vi "Read Counter Input PWM Module.vi"   [LabVIEW 2017, in "Scan Engine Scripting.lvlib"]
uses:
  Scan Engine Scripting.lvlib
  NI 9423/NI 9423.lvclass
  NI 9437/NI 9437.lvclass
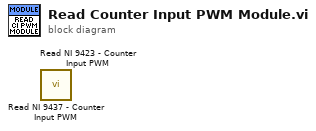
[diagram p0: block diagram]
diagram:
  n1 = call "Read NI 9437 - Counter Input PWM.vi"() -> ()  [unwired: 9 in, 3 out]
  n2 = call "Read NI 9423 - Counter Input PWM.vi"() -> ()  [unwired: 9 in, 3 out]
